vi "SetOSTime.vi"(10 "to UTC (T)":bool=TRUE, 11 "OS time":timestamp) -> (3 "return type":i8)   [LabVIEW 2020]
uses:
  kernel32.dll
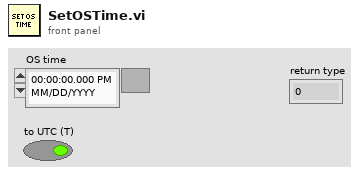
[diagram p1: front panel]
types:
  T1 = cluster{"Year":i16, "Month":i16, "Day of Week":i16, "Day of Month":i16, "Hour":i16, "Minute":i16, "Second":i16, "Millisecond":i16}
  T2 = typedef "LVDateTimeRec.ctl" = cluster{"fractional second":dbl, "second":i32, "minute":i32, "hour":i32, "day of month":i32, "month":i32, "year":i32, "day of week":i32, "day of year":i32, "DST":i32}
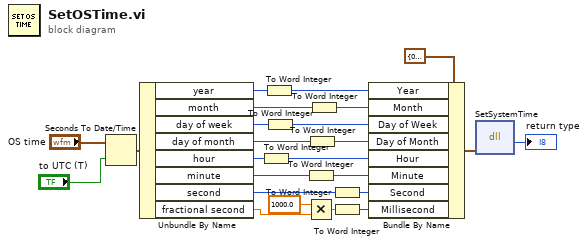
[diagram p0: block diagram]
diagram:
  n1 = Seconds To Date/Time(time stamp (now)="OS time", to UTC (F)="to UTC (T)") -> (date time rec=w19:T2)
  n2 = Unbundle By Name(w19) -> ("year"=w16:i32, "month"=w15:i32, "day of week"=w14:i32, "day of month"=w13:i32, "hour"=w12:i32, "minute"=w11:i32, "second"=w10:i32, "fractional second"=w9:dbl)
  n3 = To Word Integer(number=w12) -> (16bit integer=w3:i16)
  n4 = To Word Integer(number=w16) -> (16bit integer=w7:i16)
  n5 = To Word Integer(number=w14) -> (16bit integer=w5:i16)
  n6 = To Word Integer(number=w11) -> (16bit integer=w2:i16)
  n7 = Multiply(x=1000.0, y=w9) -> (x*y=w17:dbl)
  n8 = To Word Integer(number=w13) -> (16bit integer=w4:i16)
  n9 = To Word Integer(number=w15) -> (16bit integer=w6:i16)
  n10 = To Word Integer(number=w10) -> (16bit integer=w1:i16)
  n11 = To Word Integer(number=w17) -> (16bit integer=w8:i16)
  n12 = Bundle By Name(cluster=T1 {"Year"=0, "Month"=0, "Day of Week"=0, "Day of Month"=0, "Hour"=0, "Minute"=0, "Second"=0, "Millisecond"=0}, "Year"=w7, "Month"=w6, "Day of Week"=w5, "Day of Month"=w4, "Hour"=w3, "Minute"=w2, "Second"=w1, "Millisecond"=w8) -> (w22:T1)
  n13 = dll-call lib="kernel32.dll" fn="SetSystemTime"("time"=w22) -> ("return type"=→"return type":i8)  [unwired: 4 in, 2 out]
